vi "KundtsTube.vi"() -> ()   [LabVIEW 2015]
panel:
  out "XY Graph":cluster{"X":dbl, "Y":dbl}[](graph)
  out "RMS":dbl[](array[numeric])
  in  "Digitalizing Parameters":cluster{"Sample Rate":dbl, "# of Cycles":dbl}
  out "Waveform Graph":dynamicdata(graph)
  in  "Stop":bool
  in  "Wave Parameters":cluster{"Frequency":dbl, "Amplitude":dbl}
  in  "Sweep Controls":T1
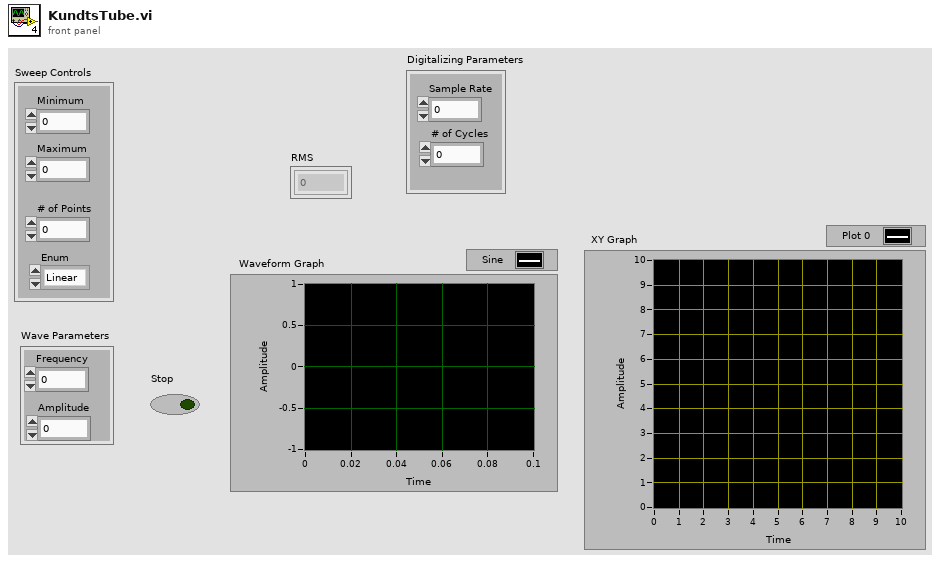
[diagram p1: front panel]
types:
  T1 = cluster{"Minimum":dbl, "Maximum":dbl, "# of Points":dbl, "Enum":enum16{"Linear", "Log10"}}
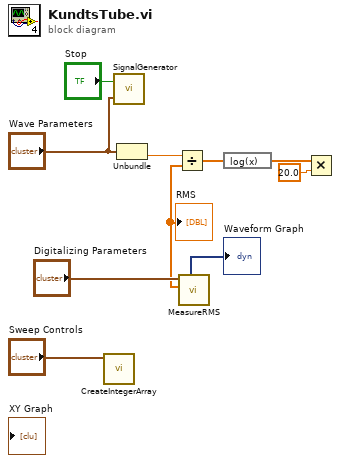
[diagram p0: block diagram]
diagram:
  n1 = call "CreateIntegerArray.vi"("Sweep Controls"="Sweep Controls") -> ()  [unwired: 10 in, 1 out]
  n2 = call "SignalGenerator.vi"("Wave Parameters"="Wave Parameters", "Stop"="Stop") -> ()  [unwired: 1 in, 1 out]
  n3 = Unbundle("Wave Parameters") -> ("Amplitude"=w1:dbl)  [unwired: 1 out]
  n4 = call "MeasureRMS.vi"("Digitalizing Parameters"="Digitalizing Parameters") -> ("Waveform Graph"=→"Waveform Graph":dynamicdata, "RMS"=w5:dbl[])  [unwired: 9 in]
  "RMS" <- w5
  n5 = Divide(x=w1, y=w5) -> (x/y=w6:dbl[])
  n6 = expression code="log(x)"(w6) -> (w3:dbl[])
  n7 = Multiply(x=w3, y=20.0) -> ()  [unwired: 1 out]
